vi "Get Consumer Values.vi"(8 "error in":errorcluster, 11 "Power Supply Cluster.lvclass in":refnum<class "Power Supply Cluster.lvclass">) -> (0 "error out":errorcluster, 1 "Consumer Ch":T1[](array[typedef]), 2 "Consumer Control":T2, 3 "Power Supply Cluster.lvclass out":refnum<class "Power Supply Cluster.lvclass">)   [LabVIEW 2023, in "Power Supply Cluster.lvclass"]
uses:
  Power Supply Cluster.lvclass
  Consumer Control.ctl
  Consumer Ch.ctl
  Power Supply Cluster.lvclass/Power Supply Cluster.ctl
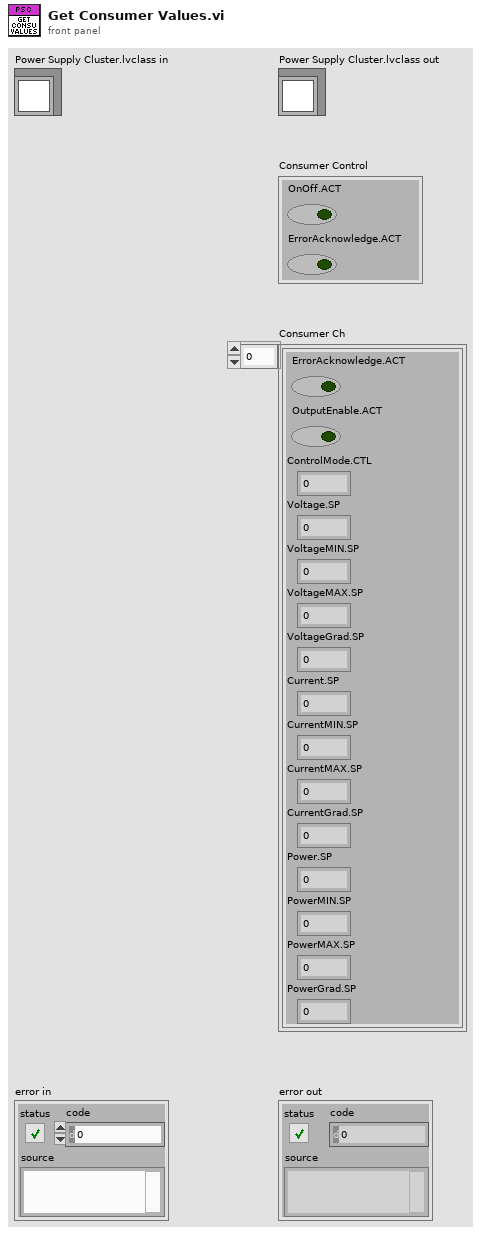
[diagram p1: front panel]
types:
  T1 = typedef "Power Supply Cluster.lvclass/Consumer Ch.ctl" = cluster{"ErrorAcknowledge.ACT":bool, "OutputEnable.ACT":bool, "ControlMode.CTL":u16, "Voltage.SP":dbl, "VoltageMIN.SP":dbl, "VoltageMAX.SP":dbl, "VoltageGrad.SP":dbl, "Current.SP":dbl, "CurrentMIN.SP":dbl, "CurrentMAX.SP":dbl, "CurrentGrad.SP":dbl, "Power.SP":dbl, "PowerMIN.SP":dbl, "PowerMAX.SP":dbl, "PowerGrad.SP":dbl}
  T2 = typedef "Power Supply Cluster.lvclass/Consumer Control.ctl" = cluster{"OnOff.ACT":bool, "ErrorAcknowledge.ACT":bool}
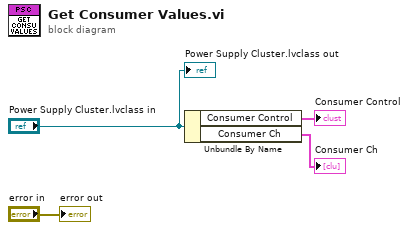
[diagram p0: block diagram]
diagram:
  n1 = Unbundle By Name("Power Supply Cluster.lvclass in") -> ("Consumer Control"=→"Consumer Control":T2, "Consumer Ch"=→"Consumer Ch":T1[])
  "error out" <- "error in"
  "Power Supply Cluster.lvclass out" <- "Power Supply Cluster.lvclass in"
